vi "config.vi"(8 "error in (no error)":errorcluster, 11 "Pistofono in":refnum<class "Pistofono.lvclass">) -> (0 "error out":errorcluster, 3 "Pistofono out":refnum<class "Pistofono.lvclass">)   [LabVIEW 2019, in "Pistofono.lvclass"]
uses:
  Pistofono.lvclass
  Pistofono.lvclass/Pistofono.ctl
  <vilib>/Instr/_visa.llb/VISA Configure Serial Port (Instr).vi
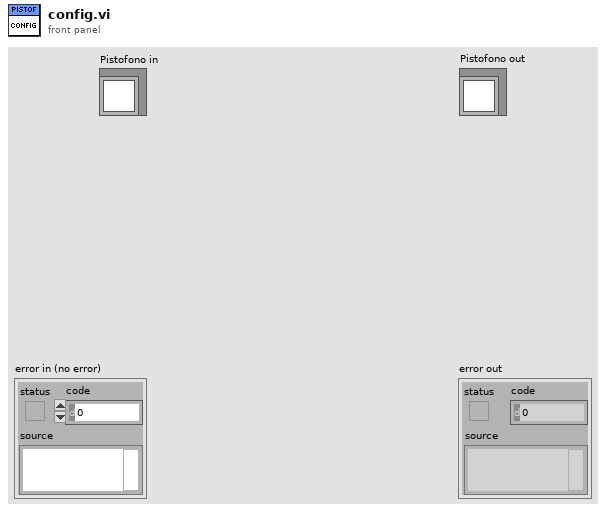
[diagram p1: front panel]
types:
  T1 = cluster{"baud rate":u32, "data bits":u16, "parity":enum16{"None", "Odd", "Even", "Mark", "Space"}, "stop bits":u16, "flow control":u16}
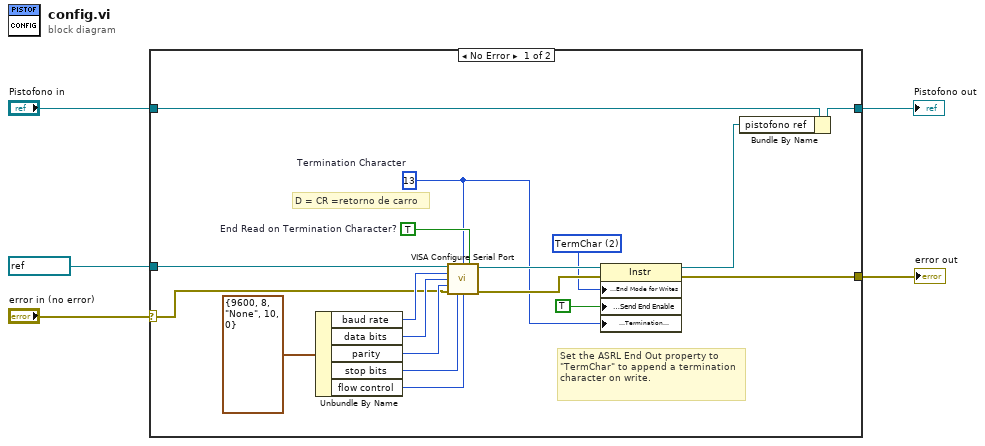
[diagram p0: block diagram]
diagram:
  n1 = case shown="No Error" "error in (no error)" {
    selector: "error in (no error)" -> [w7 w25]
    tunnel: [w6 w25] -> w4
    tunnel: [w9 w24] -> w2
    tunnel: "Pistofono in" -> [w23 w24]
    tunnel: refnum<visa-resource-name> "COM3" ("VISA resource name") -> [w10 _]
    frame No Error {
      w13 = u8 13  # Termination Character
      w12 = u16 2 items=["None", "LastBit", "TermChar", "Break"] ("Serial Settings:Serial End Mode for Writes")
      w15 = TRUE  # End Read on Termination Character?
      # "D = CR =retorno de carro"
      # "Set the ASRL End Out property to \"TermChar\" to append a termination character on write."
      n2 = Unbundle By Name(T1 {"baud rate"=9600, "data bits"=8, "parity"=enum."None", "stop bits"=10, "flow control"=0} ("Serial Settings")) -> ("baud rate"=w17:u32, "data bits"=w18:u16, "parity"=w19:enum16{"None", "Odd", "Even", "Mark", "Space"}, "stop bits"=w20:u16, "flow control"=w14:u16)
      n3 = call-poly "VISA Configure Serial Port"("VISA resource name"=w10, "termination char\n(0xA = '\\n' = LF)"=w13, "Enable Termination\nChar (T)"=w15, "baud rate (9600)"=w17, "data bits (8)"=w18, "parity (0:none)"=w19, "error in (no error)"=w7, "stop bits (10: 1 bit)"=w20, "flow control (0:none)"=w14) -> ("VISA resource name out"=w21:refnum<visa-resource-name>, "error out"=w22:errorcluster)  [unwired: 1 in, 4 out]
      n4 = property class="Instr"(reference=w21, error in=w22, "Serial Settings:End Mode for Writes"=w12, "Message Based Settings:Send End Enable"=TRUE, "Message Based Settings:Termination Character"=w13) -> (reference out=w8:refnum<visa-resource-name>, error out=w6:errorcluster)
      n5 = Bundle By Name(cluster=w23, "pistofono ref"=w8) -> (w9:refnum<class "Pistofono.lvclass">)
    }
    frame Error {
    }
  }
  "error out" <- w4
  "Pistofono out" <- w2
